vi "PID_Tuning.vi"() -> ()   [LabVIEW 2019]
uses:
  Shared VIs/ENPID/PID_Settings.ctl
  Shared VIs/ENPID/Gains.ctl
  Shared VIs/ENPID/NonLinearGainParams.ctl
  Shared VIs/ENPID/NonLinearGain.ctl
  Shared VIs/ENPID/DPartVariable.ctl
  Shared VIs/ENPID/VelocityEstimate.ctl
  Shared VIs/ENPID/OutputRange.ctl
  Shared VIs/ClusterType/RobotStateType.ctl
  Shared VIs/ModelSpecific/ETHMikeModel.ctl
  TrajectoryType.ctl
  Shared VIs/TypeDef_TDMS_States.ctl
  Shared VIs/ModelSpecific/TypeDefTachometerParam.ctl
  <vilib>/myRIO/Common/Instrument Driver Framework/myRIO v1.0/Encoder/typedefs/Encoder Signal Mode.ctl
  Shared VIs/ModelSpecific/ReadOnlyGlobalActions.ctl
  <vilib>/myRIO/Instrument Drivers/Onboard IO/AI/typedefs/AI Reference.ctl
  <vilib>/myRIO/Common/Instrument Driver Framework/Utilities/typedefs/myRIO Generic Hardware Reference.ctl
  <vilib>/myRIO/Common/Instrument Driver Framework/Utilities/typedefs/Hardware Version Enum.ctl
  <vilib>/myRIO/Common/Instrument Driver Framework/Utilities/typedefs/myRIO v1.0 Reference.ctl
  <vilib>/myRIO/Common/Instrument Driver Framework/Utilities/typedefs/Generic FPGA Reference.ctl
  <vilib>/myRIO/Common/Instrument Driver Framework/myRIO v1.0/AI/typedefs/AI Channels List.ctl
  <vilib>/myRIO/Common/Instrument Driver Framework/myRIO v1.0/AI/typedefs/AI Channels Enum.ctl
  <vilib>/myRIO/Common/Instrument Driver Framework/Utilities/typedefs/Analog Scaling Constants List.ctl
  <vilib>/myRIO/Common/Instrument Driver Framework/Utilities/typedefs/Analog Scaling Constants.ctl
  <vilib>/userDefined/High Color/nirio_resource_hc.ctl
  <vilib>/myRIO/Instrument Drivers/Onboard IO/AO/typedefs/AO Reference.ctl
  <vilib>/myRIO/Common/Instrument Driver Framework/myRIO v1.0/AO/typedefs/AO Channels List.ctl
  <vilib>/myRIO/Common/Instrument Driver Framework/myRIO v1.0/AO/typedefs/AO Channels Enum.ctl
  <vilib>/Platform/TimedLoop/XDataNode/timing_clust.ctl
  <vilib>/Platform/TimedLoop/XDataNode/nitl_modes.ctl
  <vilib>/Platform/TimedLoop/XDataNode/wakeup.ctl
  <vilib>/myRIO/Common/Instrument Driver Framework/myRIO v1.0/AI/vis/myRIO v1.1 Open AI.vi
  <vilib>/myRIO/Common/Instrument Driver Framework/myRIO v1.0/AO/vis/myRIO v1.1 Open AO.vi
  <vilib>/myRIO/Common/Instrument Driver Framework/Utilities/vis/Validate Channels.vi
  <vilib>/myRIO/Common/Instrument Driver Framework/myRIO v1.0/AI/vis/myRIO v1.0 Reserve AI.vi
  <vilib>/myRIO/Common/Instrument Driver Framework/myRIO v1.0/AO/vis/myRIO v1.0 Reserve AO.vi
  <vilib>/myRIO/Common/Instrument Driver Framework/myRIO v1.0/AO/vis/myRIO v1.0 Close AO.vi
  <vilib>/myRIO/Common/Instrument Driver Framework/myRIO v1.0/AI/vis/myRIO v1.0 Close AI.vi
  <vilib>/myRIO/Common/Instrument Driver Framework/myRIO v1.0/Encoder/vis/myRIO v1.0 Close Encoder.vi
  <vilib>/myRIO/Common/Instrument Driver Framework/myRIO v1.0/AI/vis/myRIO v1.0 Build MUX Configuration AI.vi
  <vilib>/myRIO/Common/Instrument Driver Framework/myRIO v1.0/Resource Manager/vis/myRIO v1.0 Reserve Channel List.vi
  <vilib>/myRIO/Common/Instrument Driver Framework/myRIO v1.0/AO/vis/myRIO v1.0 Build MUX Configuration AO.vi
  <vilib>/myRIO/Common/Instrument Driver Framework/myRIO v1.0/AO/vis/myRIO v1.0 Unreserve AO.vi
  <vilib>/myRIO/Common/Instrument Driver Framework/myRIO v1.0/AI/vis/myRIO v1.0 Unreserve AI.vi
  <vilib>/myRIO/Common/Instrument Driver Framework/myRIO v1.0/Encoder/vis/myRIO v1.0 Unreserve Encoder.vi
  <vilib>/myRIO/Common/Instrument Driver Framework/myRIO v1.0/Resource Manager/vis/myRIO v1.0 Reserve Channel.vi
  <vilib>/myRIO/Common/Instrument Driver Framework/myRIO v1.0/Resource Manager/vis/myRIO v1.0 Unreserve Channel.vi
  <vilib>/myRIO/Common/Instrument Driver Framework/myRIO v1.0/Resource Manager/vis/myRIO v1.0 Unreserve Channel List.vi
  <vilib>/myRIO/Common/Instrument Driver Framework/myRIO v1.0/Encoder/vis/myRIO v1.0 Build MUX Configuration Encoder.vi
  <vilib>/myRIO/Common/Instrument Driver Framework/myRIO v1.0/Resource Manager/vis/myRIO v1.0 Build Mutex Name.vi
  <vilib>/myRIO/Common/Instrument Driver Framework/myRIO v1.0/Resource Manager/vis/myRIO v1.0 Create Configuration List.vi
  <vilib>/Utility/VariantDataType/GetNumericInfo.vi
  <vilib>/Utility/error.llb/Error Cluster From Error Code.vi
  <vilib>/myRIO/Common/Instrument Driver Framework/myRIO v1.0/myRIO v1.1 Open.vi
  <vilib>/myRIO/Common/Instrument Driver Framework/myRIO v1.0/AO/vis/myRIO v1.0 Get Scaling Constants AO.vi
  <vilib>/myRIO/Common/Instrument Driver Framework/Utilities/vis/IO Manager.vi
  <vilib>/myRIO/Common/Instrument Driver Framework/Utilities/vis/Configuration Manager.vi
  <vilib>/myRIO/Common/Instrument Driver Framework/myRIO v1.0/myRIO v1.0 Close.vi
  <vilib>/myRIO/Common/Instrument Driver Framework/myRIO v1.0/AO/vis/myRIO v1.0 Write AO.vi
  <vilib>/myRIO/Common/Instrument Driver Framework/myRIO v1.0/AI/vis/myRIO v1.0 Get Scaling Constants AI.vi
  <vilib>/myRIO/Common/Instrument Driver Framework/myRIO v1.0/Encoder/vis/myRIO v1.0 Enable Encoder.vi
  <vilib>/myRIO/Common/Instrument Driver Framework/myRIO v1.0/Encoder/vis/myRIO v1.0 Shutdown Encoder.vi
  <vilib>/myRIO/Common/Instrument Driver Framework/myRIO v1.0/Resource Manager/vis/myRIO v1.0 Configure IO.vi
  <vilib>/myRIO/Instrument Drivers/Onboard IO/AO/vis/myRIO AO Open.xnode
  <vilib>/myRIO/Instrument Drivers/Onboard IO/AI/vis/myRIO AI Open.xnode
  <vilib>/platform/TimedLoop/XDataNode/XDataNode.xnode
  <vilib>/Platform/TimedLoop/XDataNode/XDNodeRunTimeDep.lvlib
  <vilib>/myRIO/Instrument Drivers/Onboard IO/AO/AO.lvlib
  <vilib>/myRIO/Instrument Drivers/Onboard IO/Encoder/Encoder.lvlib
  <vilib>/myRIO/Instrument Drivers/Onboard IO/AI/AI.lvlib
  <vilib>/addons/control/pid/NI_PID_pid.lvlib
  <vilib>/ptbypt/NI_PtbyPt.lvlib
panel:
  in  "Tachometer param":T1={"Offset [V]"=0.0, "Gain [deg/sV]"=130.0}
  out "Current Setpoint":dbl(graph)
  out "Control Output":dbl[][](graph)
  out "Control Output":cluster{"up":dbl, "ui":dbl, "ud":dbl, "u":dbl}(graph)
  out "Position Setpoint":dbl[][](graph)
  out "Velocity":cluster{"Velocity [deg/s]":dbl, dbl}(graph)
  out "Position":dbl(graph)
  out "u":cluster{"up":dbl, "ui":dbl, "ud":dbl, "u":dbl}
  out "TDMS States":T2
  in  "Trajectory Type":T3=enum."Sinus"
  in  "parameter source":T4=enum."ETH Mike #3" caption="From"
  in  "Load tuning parameter":bool caption="Boolean"
  in  "stop":bool
  out "RobotState":T5
  out "finished late":i16(graph)
  in  "PID Settings":T6={"Gains"={"K(e)"=0.0, "Kp"=0.800000011920929, "Ki"=0.0, "Kd"=0.003000000026077032}, "Non-linear gain"={"Non-linear gain P"=enum."off", "Non-linear gain I"=enum."off", "Non-linear gain D"=enum."off"}, "D-Part variable"=enum."process variable", "Velocity estimate dy/dt"=enum."external", "Anti reset windup"=TRUE, "I-Part error band"=inf, "Output range"={"output high"=0.0, "output low"=0.0}}
  in  "Target / HalfAmplitude  (deg)":dbl
  out "Current Setpoint [A]":dbl
  out "Position Setpoint [deg]":dbl
  in  "TDMS Storage File Input":string
  in  "Save data?":bool
  in  "Run":bool
  in  "Trajectory Duration (s)":dbl
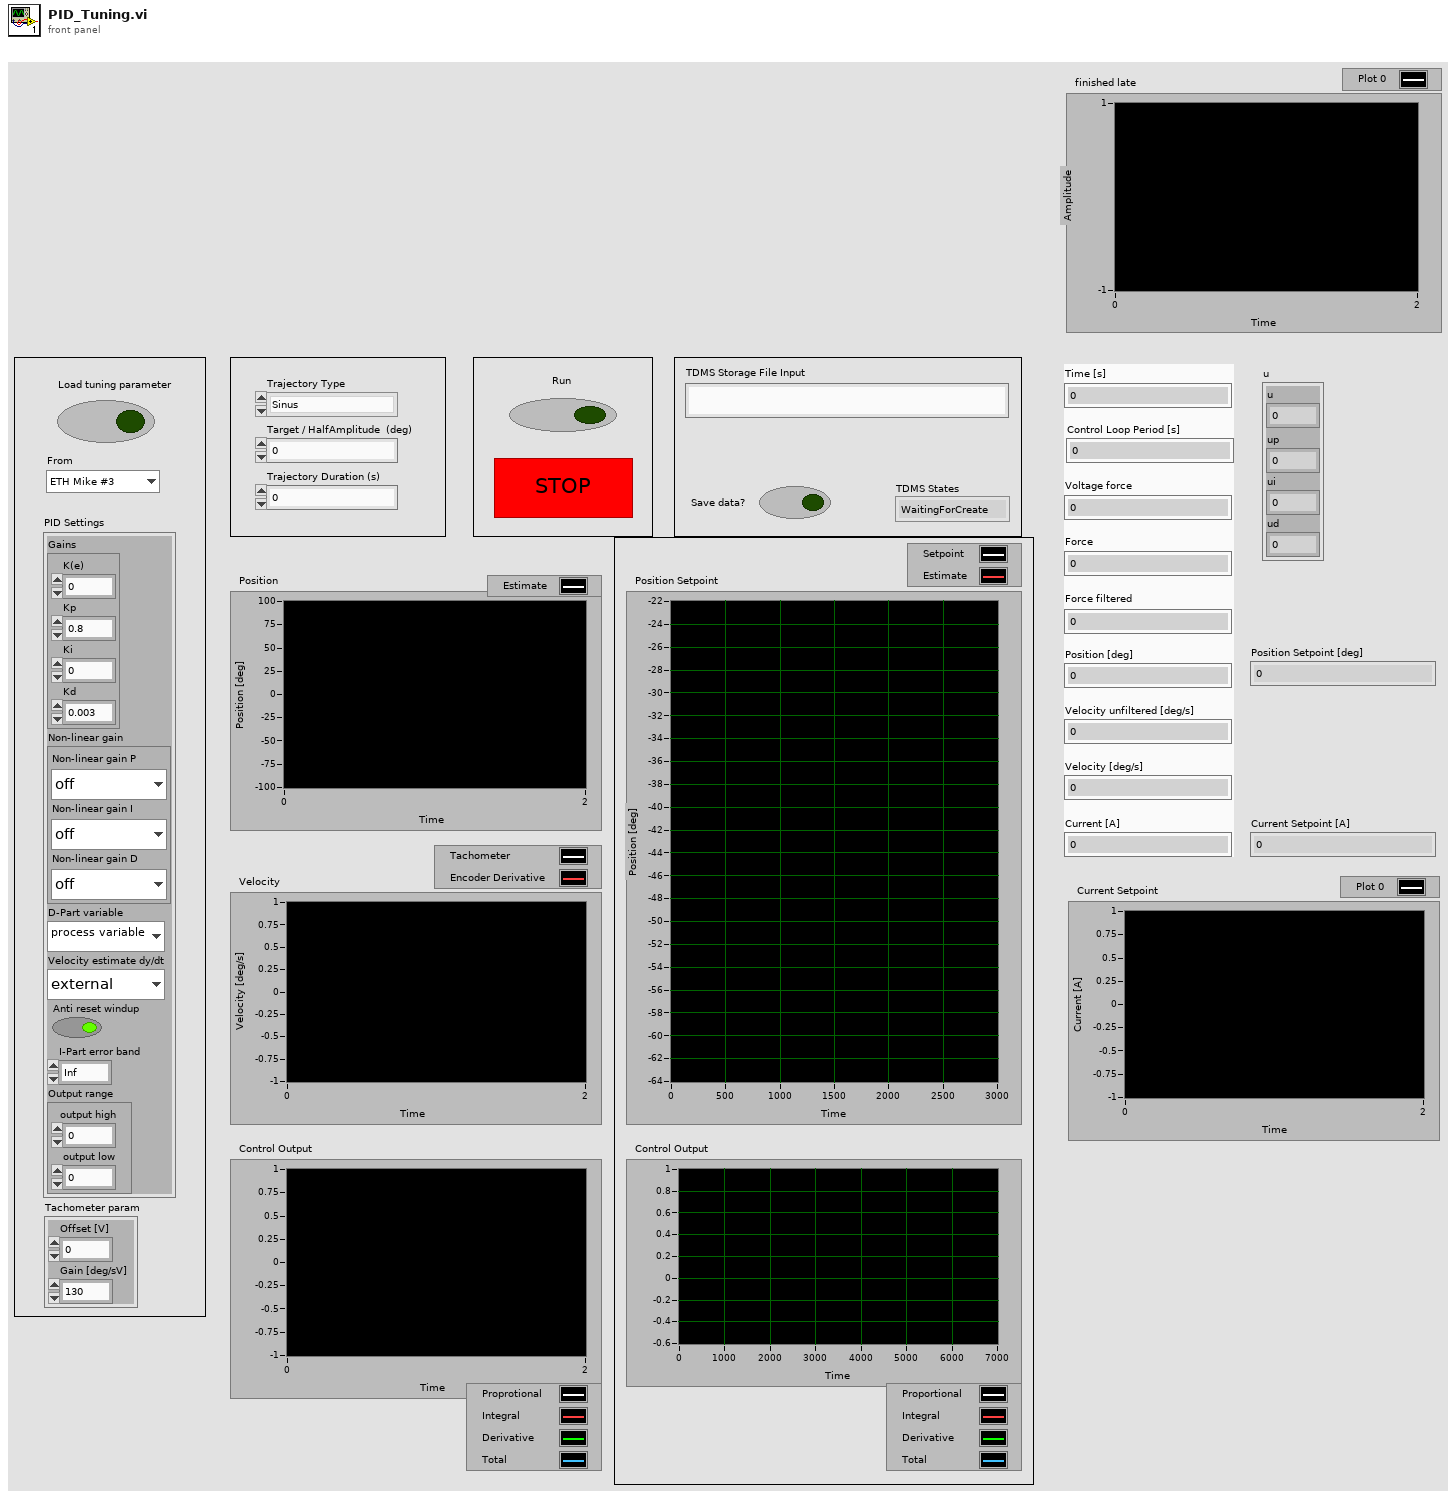
[diagram p1: front panel]
types:
  T1 = typedef "TypeDefTachometerParam.ctl" = cluster{"Offset [V]":dbl, "Gain [deg/sV]":dbl}
  T2 = typedef "TypeDef_TDMS_States.ctl" = enum16{"WaitingForCreate", "Create", "Buffering", "Flushing", "Write", "Close"}
  T3 = typedef "TrajectoryType.ctl" = enum16{"MinJerk", "Sinus", "Ramp"}
  T4 = typedef "ETHMikeModel.ctl" = enum16{"ETH Mike #1", "ETH Mike #2", "ETH Mike #3", "ETH Mike #4", "ETH MIKE #5"}
  T5 = typedef "RobotStateType.ctl" = cluster{"Time [s]":dbl, "Voltage force":dbl, "Force":dbl, "Force filtered":dbl, "Position [deg]":dbl, "Velocity unfiltered [deg/s]":dbl, "Velocity [deg/s]":dbl, "Current [A]":dbl, "Control Loop Period [s]":dbl}
  T6 = typedef "PID_Settings.ctl" = cluster{"Gains":T7, "Non-linear gain":T8, "D-Part variable":T10, "Velocity estimate dy/dt":T11, "Anti reset windup":bool, "I-Part error band":dbl, "Output range":T12}
  T7 = typedef "Gains.ctl" = cluster{"K(e)":dbl, "Kp":dbl, "Ki":dbl, "Kd":dbl}
  T8 = typedef "NonLinearGainParams.ctl" = cluster{"Non-linear gain P":T9, "Non-linear gain I":T9, "Non-linear gain D":T9}
  T9 = typedef "NonLinearGain.ctl" = enum16{"exponential", "quadratic", "off"}
  T10 = typedef "DPartVariable.ctl" = enum16{"error", "process variable"}
  T11 = typedef "VelocityEstimate.ctl" = enum16{"derivative", "external"}
  T12 = typedef "OutputRange.ctl" = cluster{"output high":dbl, "output low":dbl}
  T13 = typedef "nirio_resource_hc.ctl" = tag
  T14 = typedef "Hardware Version Enum.ctl" = enum16{"Unknown", "myRIO-1900", "myRIO-1950", "roboRIO", "NI ELVIS RIO CM", "ELVIS III"}
  T15 = enum16{"open", "open or create", "create or replace", "create", "open (read-only)"}
  T16 = typedef "XDNodeRunTimeDep.lvlib/timing_clust.ctl" = cluster{"Expected End [f-1]":u64, "Actual End [f-1]":u64, "Finished Late? [f-1]":bool, "Expected End [i-1]":u64, "Actual End [i-1]":u64, "Finished Late? [i-1]":bool, "Expected Start [i]":u64, "Actual Start [i]":u64, "Expected Start [f]":u64, "Actual Start [f]":u64, "Source Name":string, "Structure Name":string, "Period":i64, "Deadline":i64, "Offset":i64, "Start":i64, "Priority":i32, "Timeout":i32, "Mode":T17, "Wakeup Reason":T18, "Error":errorcluster, "Source Type":string, "Secondary Source Type":string, "Global End Time":u64, "Global Start Time":u64, "Frame Duration":u64, "Iteration Duration":u64, "Assigned CPU":i32, "I/O Scan Engine Mode":u32}
  T17 = typedef "XDNodeRunTimeDep.lvlib/nitl_modes.ctl" = enum32{"No Change", "Process missed periods, maintain original phase", "Discard missed periods, maintain original phase", "Process missed periods, ignore original phase", "Discard missed periods, ignore original phase"}
  T18 = typedef "XDNodeRunTimeDep.lvlib/wakeup.ctl" = enum32{"Normal", "Aborted", "Asynchronous wakeup", "Timing source error", "Timed loop error", "Timeout"}
  T19 = typedef "ReadOnlyGlobalActions.ctl" = enum16{"Initialize", "Read", "Write"}
  T20 = typedef "Encoder Signal Mode.ctl" = enum16{"Quadrature phase signal", "Step and direction signal"}
  T21 = typedef "AO.lvlib/AO Reference.ctl" = cluster{"myRIO Reference":T22, "AO Channel List":T25, "AO Scaling Constant List":T27}
  T22 = typedef "myRIO Generic Hardware Reference.ctl" = cluster{"myRIO Model":T14, "myRIO Hardware Reference":T23}
  T23 = typedef "myRIO v1.0 Reference.ctl" = cluster{"Generic FPGA Reference":T24, "Allow multiple opens":bool}
  T24 = typedef "Generic FPGA Reference.ctl" = refnum<k20>
  T25 = typedef "AO Channels List.ctl" = T26[]
  T26 = typedef "AO Channels Enum.ctl" = enum16{"Not Connected", "AudioOut/Left", "AudioOut/Right", "C/AO0", "C/AO1", "A/AO0", "A/AO1", "B/AO0", "B/AO1"}
  T27 = typedef "Analog Scaling Constants List.ctl" = T28[]
  T28 = typedef "Analog Scaling Constants.ctl" = cluster{"LSB Weight (Volts)":dbl, "Offset (Volts)":dbl, "Signed?":bool}
  T29 = typedef "Encoder.lvlib/Encoder Reference.ctl" = cluster{"myRIO Reference":T22, "Encoder Channels Enum":T30}
  T30 = typedef "Encoder Channels Enum.ctl" = enum16{"Not Connected", "C/ENC0", "C/ENC1", "A/ENC", "A/ENC0", "A/ENC1", "A/ENC2", "A/ENC3", "A/ENC4", "A/ENC5", "A/ENC6", "A/ENC7", "A/ENC8", "A/ENC9", "B/ENC", "B/ENC0", "B/ENC1", "B/ENC2", "B/ENC3", "B/ENC4", "B/ENC5", "B/ENC6", "B/ENC7", "B/ENC8", "B/ENC9", "DIO/ENC0", "DIO/ENC1", "DIO/ENC2", "DIO/ENC3", "DIO/ENC4"}
  T31 = typedef "AI.lvlib/AI Reference.ctl" = cluster{"myRIO Reference":T22, "AI Channels List":T32, "AI Scaling Constants List":T27}
  T32 = typedef "AI Channels List.ctl" = T33[]
  T33 = typedef "AI Channels Enum.ctl" = enum16{"Not Connected", "AudioIn/Left", "AudioIn/Right", "C/AI0", "C/AI1", "A/AI0", "A/AI1", "A/AI2", "A/AI3", "A/AI4", "A/AI5", "A/AI6", "A/AI7", "B/AI0", "B/AI1", "B/AI2", "B/AI3", "B/AI4", "B/AI5", "B/AI6", "B/AI7", "AI/AI0", "AI/AI1", "AI/AI2", "AI/AI3", "A/AI0 (DIFF)", "A/AI1 (DIFF)", "A/AI2 (DIFF)", "A/AI3 (DIFF)", "B/AI0 (DIFF)", "B/AI1 (DIFF)", "B/AI2 (DIFF)", "B/AI3 (DIFF)"}
  T34 = cluster{"Encoder":T29, "Tachometer":T31, "Motor Current Monitor":T31, "Force Sensor":T31}
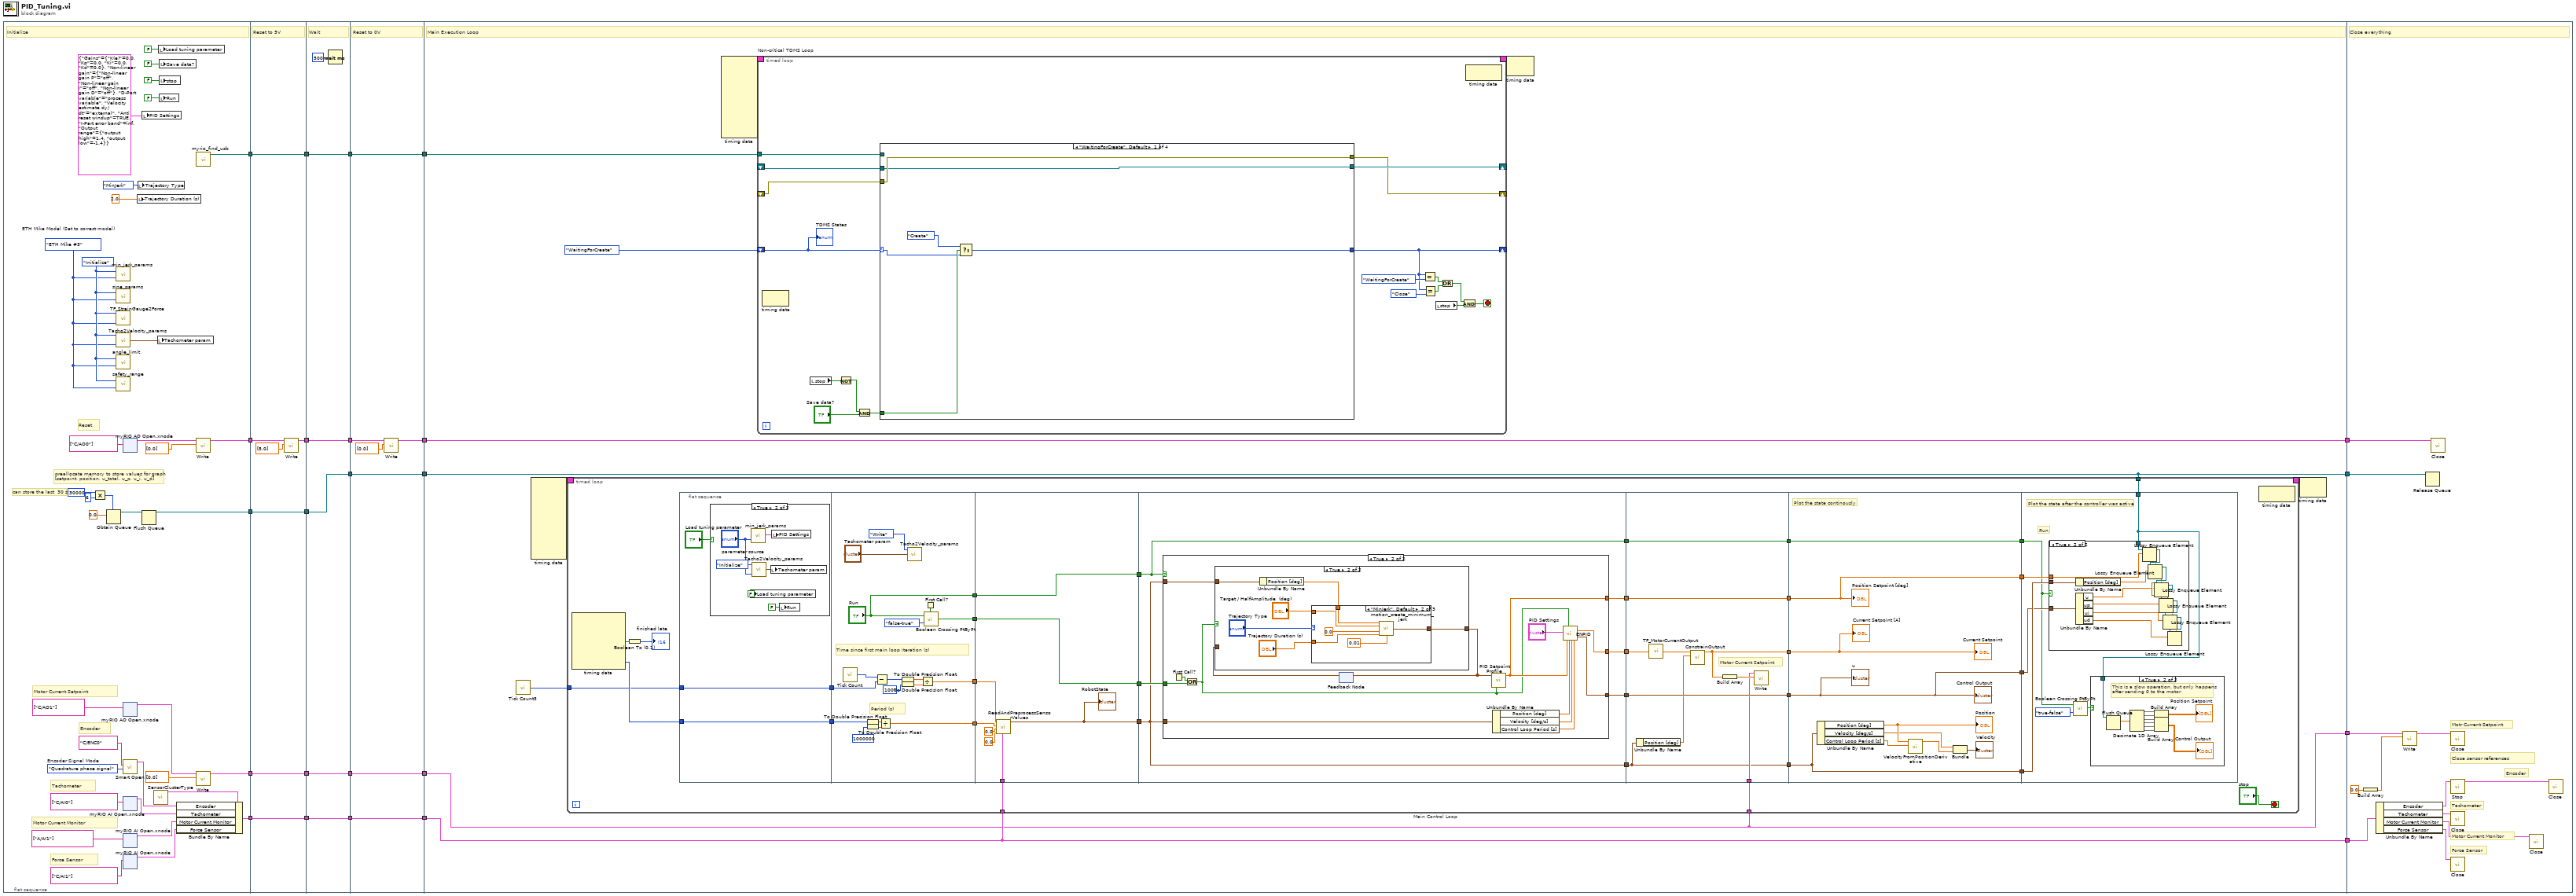
[diagram p0: block diagram]
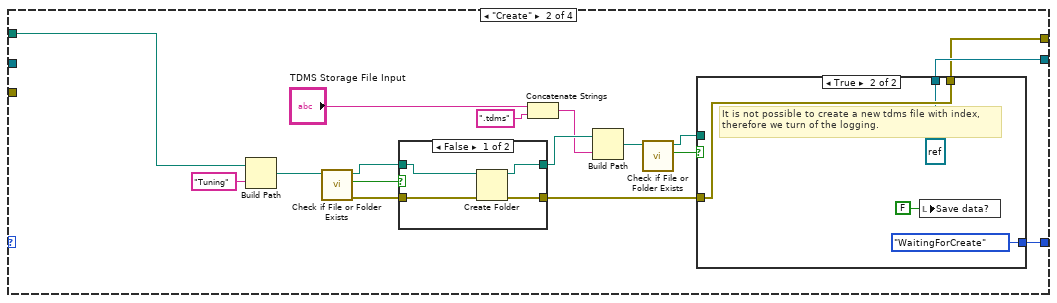
[diagram p2: hidden frame]
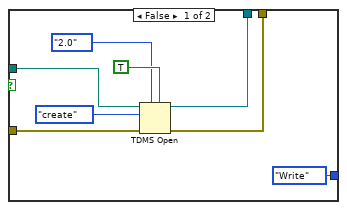
[diagram p3: hidden frame]
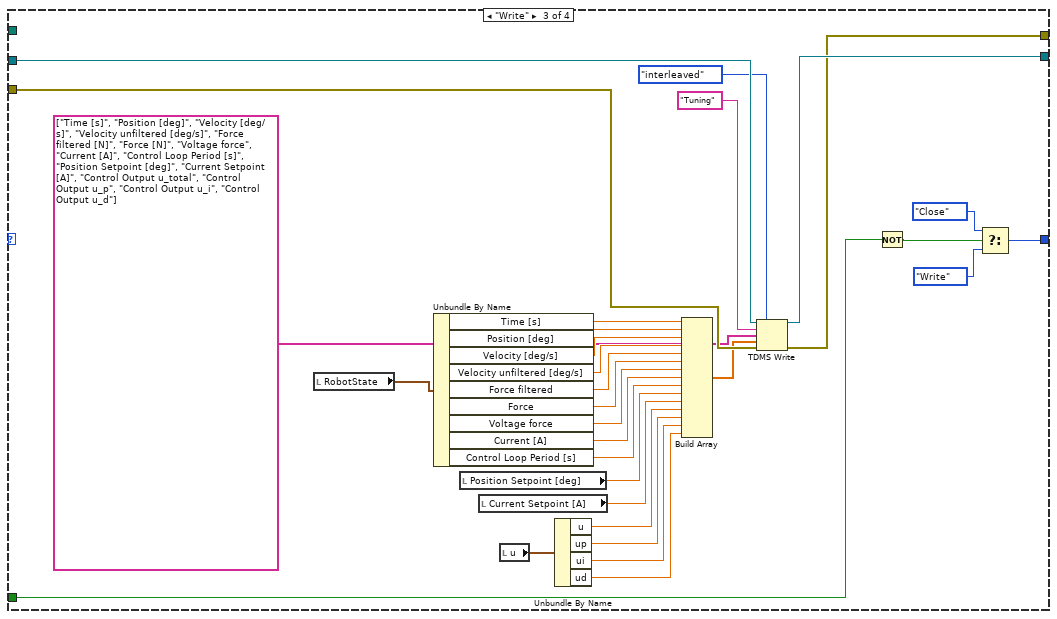
[diagram p5: hidden frame]
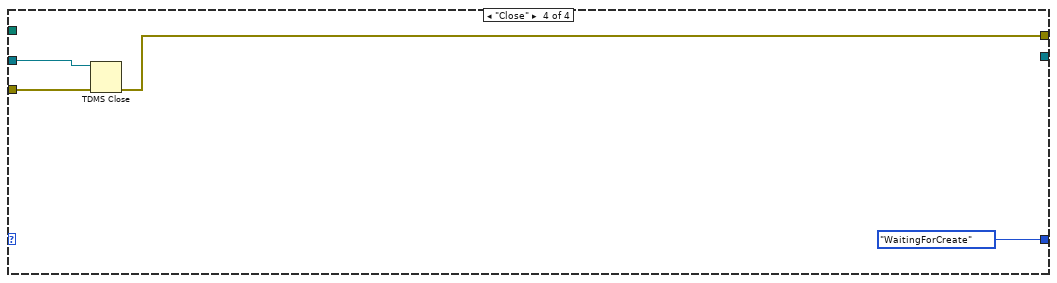
[diagram p6: hidden frame]
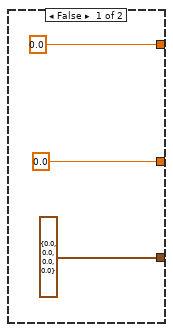
[diagram p8: hidden frame]
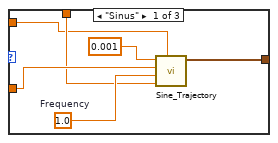
[diagram p10: hidden frame]
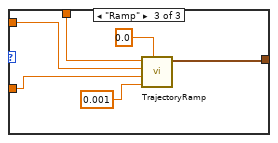
[diagram p11: hidden frame]
diagram:
  n1 = flat-sequence {
    tunnel: [w57] -> w24
    tunnel: [w53] -> w17
    tunnel: [w42] -> w13
    tunnel: [w41] -> w12
    tunnel: [w29] -> w2
    tunnel: w24 -> [w156]
    tunnel: [w155] -> w23
    tunnel: [w154] -> w18
    tunnel: w17 -> [w154]
    tunnel: [w153] -> w14
    tunnel: w13 -> [w153]
    tunnel: w12 -> [w152]
    tunnel: [w152] -> w11
    tunnel: [w151] -> w3
    tunnel: w2 -> [w151]
    tunnel: w23 -> [w163]
    tunnel: [w163] -> w22
    tunnel: [w161] -> w19
    tunnel: w18 -> [w161]
    tunnel: [w160] -> w15
    tunnel: w14 -> [w160]
    tunnel: w11 -> [w159]
    tunnel: [w159] -> w10
    tunnel: [w158] -> w4
    tunnel: w3 -> [w158]
    tunnel: w22 -> [w169]
    tunnel: [w168] -> w21
    tunnel: [w167] -> w20
    tunnel: w19 -> [w167]
    tunnel: [w166] -> w16
    tunnel: w15 -> [w166]
    tunnel: w10 -> [w165]
    tunnel: [w165] -> w9
    tunnel: [w164] -> w5
    tunnel: w4 -> [w164]
    tunnel: w21 -> [w178]
    tunnel: w20 -> [w179]
    tunnel: w16 -> [w176]
    tunnel: w9 -> [w175]
    tunnel: [w175] -> w8
    tunnel: [w176] -> w7
    tunnel: [w178] -> w6
    tunnel: w5 -> [w171]
    tunnel: [w171] -> w1
    tunnel: w8 -> [w463]
    tunnel: w7 -> [w457]
    tunnel: w6 -> [w456]
    tunnel: w1 -> [w455]
    frame #0 {
      w40 = ReadOnlyGlobalActions."Initialize" ("Action (Read)")
      w39 = ETHMikeModel."ETH Mike #3"  # ETH Mike Model (Set to correct model)
      w51 = Encoder_Signal_Mode."Quadrature phase signal"  # Encoder Signal Mode
      # "can store the last  30 s"
      # "preallocate memory to store values for graph\n[setpoint, position, u_total, u_p, u_i, u_d]"
      # "Force Sensor"
      # "Tachometer"
      # "Motor Current Monitor"
      # "Encoder"
      # "Motor Current Setpoint"
      # "Reset"
      # "Initialize"
      n2 = Multiply(x=30000 ("max queue size (-1, unlimited)"), y=6) -> (x*y=w26:i32)
      n3 = Obtain Queue(max queue size (-1, unlimited)=w26, element data type=0.0) -> (queue out=w30:refnum<queue>)  [unwired: 3 in, 2 out]
      n4 = call "min_jerk_params.vi"("Action (Read)"=w40, "ETH Mike Model"=w39) -> ()  [unwired: 17 in, 1 out]
      n5 = call "sine_params.vi"("Action (Read)"=w40, "ETH Mike Model"=w39) -> ()  [unwired: 17 in, 1 out]
      n6 = call "TF_StrainGauge2Force.vi"("Action (Read)"=w40, "ETH Mike Model"=w39) -> ()  [unwired: 3 in, 1 out]
      n7 = call "Tacho2Velocity_params.vi"("Action (Read)"=w40, "ETH Mike Model"=w39) -> ("Cluster"=w32:T1)  [unwired: 3 in]
      n8 = call "angle_limit.vi"("ETH Mike Model"=w39, "Action (Read)"=w40) -> ()  [unwired: 1 out]
      n9 = call "safety_range.vi"("ETH Mike Model"=w39, "Action (Read)"=w40) -> ()  [unwired: 1 out]
      n10 = xnode "myRIO AO Open.xnode"("Channel Names"=tag[] ["C/AO0"]) -> ("AO Ref Out"=w59:T21)  [unwired: 2 in, 1 out]
      n11 = xnode "myRIO AO Open.xnode"("Channel Names"=tag[] ["C/AO1"]) -> ("AO Ref Out"=w55:T21)  [unwired: 2 in, 1 out]
      n12 = call <vilib>:"Smart Open.vi"("Encoder Signal Mode"=w51, "Channel Name"=tag "C/ENC0") -> ("Encoder Ref Out"=w46:T29)  [unwired: 8 in, 1 out]
      n13 = xnode "myRIO AI Open.xnode"("Channel Names"=tag[] ["C/AI0"]) -> ("AI Ref Out"=w45:T31)  [unwired: 2 in, 1 out]
      n14 = xnode "myRIO AI Open.xnode"("Channel Names"=tag[] ["A/AI1"]) -> ("AI Ref Out"=w44:T31)  [unwired: 2 in, 1 out]
      n15 = xnode "myRIO AI Open.xnode"("Channel Names"=tag[] ["C/AI1"]) -> ("AI Ref Out"=w43:T31)  [unwired: 2 in, 1 out]
      n16 = local write "Trajectory Duration (s)"(2.0 ("Ramp Duration (s)")) -> ()
      n17 = local write "Trajectory Type"(TrajectoryType."MinJerk" ("Trajectory Type")) -> ()
      n18 = local write "PID Settings"(T6 {"Gains"={"K(e)"=0.0, "Kp"=0.0, "Ki"=0.0, "Kd"=0.0}, "Non-linear gain"={"Non-linear gain P"=enum."off", "Non-linear gain I"=enum."off", "Non-linear gain D"=enum."off"}, "D-Part variable"=enum."process variable", "Velocity estimate dy/dt"=enum."external", "Anti reset windup"=TRUE, "I-Part error band"=inf, "Output range"={"output high"=1.4, "output low"=-1.4}} ("PID Settings")) -> ()
      n19 = Flush Queue(queue=w30) -> (queue out=w29:refnum<queue>)  [unwired: 1 in, 2 out]
      n20 = call "SensorClusterType.vi"() -> ("Cluster"=w47:T34)  [unwired: 11 in]
      n21 = local write "Tachometer param"(w32) -> ()
      n22 = local write "Load tuning parameter"(FALSE ("Load tuning parameter")) -> ()
      n23 = local write "Save data?"(FALSE ("Save data?")) -> ()
      n24 = local write "stop"(FALSE ("stop")) -> ()
      n25 = local write "Run"(FALSE ("Run")) -> ()
      n26 = Bundle By Name(cluster=w47, "Encoder"=w46, "Tachometer"=w45, "Motor Current Monitor"=w44, "Force Sensor"=w43) -> (w42:T34)
      n27 = call <vilib>:"Write.vi"("Values"=dbl[] [0.0], "AO Ref In"=w59) -> ("AO Ref Out"=w57:T21)  [unwired: 7 in, 1 out]
      n28 = call <vilib>:"Write.vi"("Values"=dbl[] [0.0], "AO Ref In"=w55) -> ("AO Ref Out"=w41:T21)  [unwired: 7 in, 1 out]
      n29 = call "myrio_find_usb.vi"() -> ("Largest USB Partition Path"=w53:path)  [unwired: 9 in, 2 out]
    }
    frame #1 {
      # "Reset to 5V"
      n30 = call <vilib>:"Write.vi"("Values"=dbl[] [5.0], "AO Ref In"=w156) -> ("AO Ref Out"=w155:T21)  [unwired: 7 in, 1 out]
    }
    frame #2 {
      # "Wait"
      n31 = Wait (ms)(milliseconds to wait=500) -> ()  [unwired: 1 out]
    }
    frame #3 {
      # "Reset to 0V"
      n32 = call <vilib>:"Write.vi"("Values"=dbl[] [0.0], "AO Ref In"=w169) -> ("AO Ref Out"=w168:T21)  [unwired: 7 in, 1 out]
    }
    frame #4 {
      # "Main Execution Loop"
      n33 = call "Tick Count3"() -> ("Tick Count(mSec)"=w177:u32)
      n34 = node-c288() -> (w181:T16)  [unwired: 10 in]
      n35 = timed-loop "Main Control Loop" {
        timing: w181 -> [_]
        timing-out: [_] -> w180
        tunnel: w177 -> [w301]
        tunnel: w176 -> [w298]
        tunnel: w175 -> [w280]
        tunnel: w171 -> [w279]
        stop <- "stop" stop-if-true
        n36 = node-c288() -> (w308:bool, w302:i64)  [unwired: 1 in, 5 out]
        n37 = Boolean To (0,1)(Boolean=w308) -> (0, 1=→"finished late":i16)
        n38 = flat-sequence {
          tunnel: w301 -> [w311]
          tunnel: w302 -> [w312]
          tunnel: [w312] -> w296
          tunnel: [w311] -> w295
          tunnel: [w322] -> w307
          tunnel: ["Run"] -> w306
          tunnel: [w333] -> w303
          tunnel: [w325] -> w300
          tunnel: w296 -> [w327]
          tunnel: w295 -> [w326]
          tunnel: [w343] -> w305
          tunnel: [w344] -> w304
          tunnel: w307 -> [w343]
          tunnel: w306 -> [w344]
          tunnel: w298 -> [w342]
          tunnel: w303 -> [w339]
          tunnel: w300 -> [w338]
          tunnel: [w337] -> w299
          tunnel: [w349] -> w290
          tunnel: w305 -> [w350]
          tunnel: w304 -> [w345]
          tunnel: [w348] -> w289
          tunnel: w299 -> [w348]
          tunnel: [w347] -> w287
          tunnel: [w346] -> w285
          tunnel: [w345] -> w283
          tunnel: w290 -> [w399]
          tunnel: w289 -> [w395]
          tunnel: [w395] -> w288
          tunnel: w287 -> [w402]
          tunnel: [w402] -> w286
          tunnel: w285 -> [w401]
          tunnel: [w401] -> w284
          tunnel: w283 -> [w400]
          tunnel: [w400] -> w282
          tunnel: [w393] -> w281
          tunnel: w280 -> [w396]
          tunnel: w288 -> [w410]
          tunnel: w286 -> [w411]
          tunnel: w284 -> [w405]
          tunnel: w282 -> [w412]
          tunnel: [w412] -> w294
          tunnel: [w411] -> w293
          tunnel: [w410] -> w292
          tunnel: [w405] -> w291
          tunnel: w281 -> [w406]
          tunnel: w291 -> [w415]
          tunnel: w292 -> [w417]
          tunnel: w293 -> [w418]
          tunnel: w294 -> [w414]
          tunnel: w279 -> [w413]
          frame #0 {
            n39 = case shown="True" "Load tuning parameter" {
              frame False {
              }
              frame True {
                n40 = local write "Load tuning parameter"(FALSE ("Load parameter")) -> ()
                n41 = call "min_jerk_params.vi"("ETH Mike Model"="parameter source") -> ("PID Settings"=w316:T6)  [unwired: 18 in]
                n42 = call "Tacho2Velocity_params.vi"("Action (Read)"=ReadOnlyGlobalActions."Initialize", "ETH Mike Model"="parameter source") -> ("Cluster"=w314:T1)  [unwired: 3 in]
                n43 = local write "Tachometer param"(w314) -> ()
                n44 = local write "PID Settings"(w316) -> ()
                n45 = local write "Run"(FALSE ("Run")) -> ()
              }
            }
          }
          frame #1 {
            # "Time since first main loop iteration (s)"
            # "Period (s)"
            n46 = call "Tick Count"() -> ("Tick Count(mSec)"=w328:u32)
            n47 = To Double Precision Float(number=w327) -> (double precision float=w334:dbl)
            n48 = To Double Precision Float(number=1000000) -> (double precision float=w335:dbl)
            n49 = Subtract(x=w328, y=w326) -> (x-y=w331:u32)
            n50 = Divide(x=w334, y=w335) -> (x/y=w333:dbl)
            n51 = To Double Precision Float(number=w331) -> (double precision float=w329:dbl)
            n52 = To Double Precision Float(number=u32 1000 ("y")) -> (double precision float=w330:dbl)
            n53 = call "Tacho2Velocity_params.vi"("Action (Read)"=ReadOnlyGlobalActions."Write", "Tachometer param input"="Tachometer param") -> ()  [unwired: 3 in, 1 out]
            n54 = Divide(x=w329, y=w330) -> (x/y=w325:dbl)
            n55 = First Call?() -> (First Call?: T/F=w320:bool)
            n56 = call <vilib>:"Boolean Crossing PtByPt.vi"("initialize"=w320, "direction"=enum16{"either", "false-true", "true-false"}."false-true", "input"="Run") -> ("crossing"=w322:bool)
          }
          frame #2 {
            n57 = call "ReadAndPreprocessSensorValues.vi"("Sensor References"=w342, "Force_calib_value"=0.0, "Velocity_calib_value"=0.0, "Control Loop Period [s]"=w339, "Time [s]"=w338) -> ("RobotStateType"=w337:T5)  [unwired: 6 in]
            "RobotState" <- w337
          }
          frame #3 {
            n58 = case shown="True" w345 {
              tunnel: w350 -> [_ w364]
              tunnel: [0.0 ("u") w355] -> w349
              tunnel: w348 -> [_ w363]
              tunnel: w348 -> [_ w359]
              tunnel: [0.0 ("setpoint") w357] -> w347
              tunnel: [cluster{"up":dbl, "ui":dbl, "ud":dbl, "u":dbl} {"up"=0.0, "ui"=0.0, "ud"=0.0, "u"=0.0} ("u") w354] -> w346
              frame False {
              }
              frame True {
                n59 = First Call?() -> (First Call?: T/F=w365:bool)
                n60 = Or(x=w365, y=w364) -> (x .or. y?=w356:bool)
                n61 = feedback #1() -> (w366:cluster{"time (s)":dbl, "setpoint":dbl}[])  [unwired: 1 in]
                n62 = case shown="True" w356 {
                  tunnel: [w368 w374] -> w367
                  tunnel: w366 -> [w368 _]
                  tunnel: w359 -> [_ w371]
                  frame False {
                  }
                  frame True {
                    n63 = Unbundle By Name(w371) -> ("Position [deg]"=w370:dbl)
                    n64 = case shown="\"MinJerk\", Default" "Trajectory Type" {
                      tunnel: [w377 w386 w392] -> w374
                      tunnel: "Trajectory Duration (s)" -> [w378 w383 w391]
                      tunnel: "Target / HalfAmplitude  (deg)" -> [w375 w382 w390]
                      tunnel: w370 -> [w376 w381 w389]
                      frame "Sinus" {
                        w379 = 1.0  # Frequency
                        n65 = call "Sine_Trajectory.vi"("Amplitude"=w375, "Middle Position"=w376, "Cycles"=w379, "Duration (s)"=w378, "Sampling Period (s)"=0.001) -> ("Profile"=w377:cluster{"time (s)":dbl, "setpoint":dbl}[])  [unwired: 6 in]
                      }
                      frame "MinJerk", Default {
                        n66 = call "motion_create_minimum_jerk.vi"("Initial Position"=w381, "Final Position"=w382, "Initial Time [s]"=0.0, "Final Time [s]"=w383, "Delta Time [s]"=0.01) -> ("Profile"=w386:cluster{"time (s)":dbl, "setpoint":dbl}[])  [unwired: 10 in]
                      }
                      frame "Ramp" {
                        n67 = call "TrajectoryRamp.vi"("Initial Time (s)"=0.0, "Period (s)"=0.001, "Ramp Duration (s)"=w391, "Final Position (deg)"=w390, "Initial Position (deg)"=w389) -> ("Profile 2"=w392:cluster{"time (s)":dbl, "setpoint":dbl}[])  [unwired: 6 in]
                      }
                    }
                  }
                }
                n68 = feedback-in #1(w367) -> ()
                n69 = call <vilib>:"PID Setpoint Profile.vi"("reinitialize? (F)"=w356, "setpoint profile"=w367) -> ("setpoint"=w357:dbl)  [unwired: 4 in, 3 out]
                n70 = Unbundle By Name(w363) -> ("Position [deg]"=w362:dbl, "Velocity [deg/s]"=w361:dbl, "Control Loop Period [s]"=w360:dbl)
                n71 = call "ENPID.vi"("PID Settings"="PID Settings", "r"=w357, "Reset?"=w356, "y"=w362, "dy/dt"=w361, "dt (s)"=w360) -> (15:"u"=w355:dbl, 18:"u"=w354:cluster{"u":dbl, "up":dbl, "ui":dbl, "ud":dbl})  [unwired: 12 in]
              }
            }
          }
          frame #4 {
            # "Motor Current Setpoint"
            n72 = Unbundle By Name(w395) -> ("Position [deg]"=w394:dbl)
            n73 = call "TF_MotorCurrentOutput.vi"("Motor Current Setpoint [A]"=w399) -> ("Motor Current Setpoint [V]"=w398:dbl)
            n74 = call "ConstrainOutput.vi"("Position [deg]"=w394, "Motor Current Setpoint [V]"=w398) -> ("Motor Output"=w393:dbl)  [unwired: 9 in]
            n75 = Build Array(w393) -> (w397:dbl[])
            n76 = call <vilib>:"Write.vi"("Values"=w397, "AO Ref In"=w396) -> ()  [unwired: 7 in, 2 out]
          }
          frame #5 {
            # "Plot the state continously"
            n77 = Unbundle By Name(w410) -> ("Position [deg]"=w409:dbl, "Velocity [deg/s]"=w407:dbl, "Control Loop Period [s]"=w403:dbl)
            "Position" <- w409
            n78 = call "VelocityFromPositionDerivative.vi"("Control Loop Period [s]"=w403, "Position [deg]"=w409) -> ("Velocity"=w404:dbl)  [unwired: 9 in]
            n79 = Bundle("Velocity [deg/s]"=w407, "Velocity"=w404) -> (→"Velocity":cluster{"Velocity [deg/s]":dbl, "Velocity":dbl})  [unwired: 1 in]
            "Current Setpoint [A]" <- w406
            "Position Setpoint [deg]" <- w411
            "u" <- w405
            "Control Output" <- w405
            "Current Setpoint" <- w406
          }
          frame #6 {
            # "Plot the state after the controller was active"
            # "Run"
            n80 = case shown="True" w414 {
              tunnel: w418 -> [_ w435]
              tunnel: w417 -> [_ w438]
              tunnel: w415 -> [_ w437]
              tunnel: w413 -> [_ w436]
              frame False {
              }
              frame True {
                n81 = Unbundle By Name(w438) -> ("Position [deg]"=w429:dbl)
                n82 = Unbundle By Name(w437) -> ("u"=w423:dbl, "up"=w422:dbl, "ui"=w421:dbl, "ud"=w420:dbl)
                n83 = Lossy Enqueue Element(queue=w436, element=w435) -> (queue out=w434:refnum<queue>, error out=w428:errorcluster)  [unwired: 1 in, 2 out]
                n84 = Lossy Enqueue Element(queue=w434, element=w429, error in (no error)=w428) -> (queue out=w433:refnum<queue>, error out=w427:errorcluster)  [unwired: 2 out]
                n85 = Lossy Enqueue Element(queue=w433, element=w423, error in (no error)=w427) -> (queue out=w432:refnum<queue>, error out=w426:errorcluster)  [unwired: 2 out]
                n86 = Lossy Enqueue Element(queue=w432, element=w422, error in (no error)=w426) -> (queue out=w431:refnum<queue>, error out=w425:errorcluster)  [unwired: 2 out]
                n87 = Lossy Enqueue Element(queue=w431, element=w421, error in (no error)=w425) -> (queue out=w430:refnum<queue>, error out=w424:errorcluster)  [unwired: 2 out]
                n88 = Lossy Enqueue Element(queue=w430, element=w420, error in (no error)=w424) -> ()  [unwired: 4 out]
              }
            }
            n89 = call <vilib>:"Boolean Crossing PtByPt.vi"("direction"=enum16{"either", "false-true", "true-false"}."true-false", "input"=w414) -> ("crossing"=w419:bool)  [unwired: 1 in]
            n90 = case shown="True" w419 {
              tunnel: w413 -> [_ w448]
              frame False {
              }
              frame True {
                # "This is a slow operation, but only happens\nafter sending 0 to the motor"
                n91 = Flush Queue(queue=w448) -> (remaining elements=w445:dbl[])  [unwired: 1 in, 2 out]
                n92 = Decimate 1D Array(w445) -> (w447:dbl[], w446:dbl[], w443:dbl[], w442:dbl[], w441:dbl[], w440:dbl[])
                n93 = Build Array(w447, w446) -> (→"Position Setpoint":dbl[][])
                n94 = Build Array(w443, w442, w441, w440) -> (→"Control Output":dbl[][])
              }
            }
          }
        }
        n95 = node-c288() -> ()  [unwired: 1 in, 1 out]
      }
      n96 = node-c288() -> (w174:T16)  [unwired: 10 in]
      n97 = timed-loop "Non-critical TDMS Loop" {
        timing: w174 -> [_]
        timing-out: [_] -> w173
        shift-right: [w191] -> _
        shift-left: TypeDef_TDMS_States."WaitingForCreate" ("TDMS States") -> [w194]
        tunnel: w179 -> [w199]
        shift-right: [w198] -> _
        shift-left: _ -> [w195]
        shift-right: [w197] -> _
        shift-left: _ -> [w196]
        stop <- w188 stop-if-true
        n98 = node-c288() -> ()  [unwired: 1 in, 1 out]
        n99 = local read "stop"() -> (w183:bool)
        n100 = Not(x=w183) -> (.not. x?=w182:bool)
        n101 = And(x=w182, y="Save data?") -> (x .and. y?=w185:bool)
        n102 = case shown="\"WaitingForCreate\", Default" w194 {
          selector: w194 -> [w203 _ _ _]
          tunnel: w185 -> [w205 _ w266 _]
          tunnel: [w202 w222 w267 TypeDef_TDMS_States."WaitingForCreate" ("TDMS States")] -> w191
          tunnel: w199 -> [_ w208 _ _]
          tunnel: [w200 w221 w268 _] -> w198
          tunnel: [w201 w220 w247 w272] -> w197
          tunnel: w196 -> [w201 _ w270 w273]
          tunnel: w195 -> [w200 _ w269 w274]
          frame "WaitingForCreate", Default {
            n103 = Select(t=TypeDef_TDMS_States."Create" ("TDMS States"), s=w205, f=w203) -> (s? t:f=w202:T2)
          }
          frame "Create" {
            n104 = Build Path(base path=w208, name or relative path="Tuning") -> (appended path=w207:path)
            n105 = call <vilib>:"Check if File or Folder Exists.vi"("path"=w207) -> ("error out"=w217:errorcluster, "file or folder exists?"=w219:bool, "dup path"=w218:path)  [unwired: 8 in]
            n106 = case shown="False" w219 {
              tunnel: w218 -> [w238 w239]
              tunnel: [w237 w240] -> w212
              tunnel: w217 -> [w236 w240]
              tunnel: [w235 w239] -> w216
              frame False {
                n107 = Create Folder(path (use dialog)=w238, error in=w236) -> (created path=w235:path, error out=w237:errorcluster)  [unwired: 1 in, 1 out]
              }
              frame True {
              }
            }
            n108 = Concatenate Strings("TDMS Storage File Input", ".tdms") -> (w213:string)
            n109 = Build Path(base path=w216, name or relative path=w213) -> (appended path=w211:path)
            n110 = call <vilib>:"Check if File or Folder Exists.vi"("path"=w211) -> ("file or folder exists?"=w210:bool, "dup path"=w209:path)  [unwired: 8 in, 1 out]
            n111 = case shown="True" w210 {
              tunnel: [TypeDef_TDMS_States."Write" ("TDMS States") TypeDef_TDMS_States."WaitingForCreate" ("TDMS States")] -> w222
              tunnel: [w229 refnum<k34> refnum ("tdms file out")] -> w221
              tunnel: [w228 w232] -> w220
              tunnel: w212 -> [w224 w232]
              tunnel: w209 -> [w223 _]
              frame False {
                n112 = TDMS Open(5:TRUE, 7:enum16{"1.0", "2.0"}."2.0" ("file format version (2.0)"), 8:w224, 10:T15."create" ("operation (0:open)"), 11:w223) -> (0:w228:errorcluster, 3:w229:refnum<k34>)  [unwired: 2 in]
              }
              frame True {
                # "It is not possible to create a new tdms file with index,\ntherefore we turn of the logging."
                n113 = local write "Save data?"(FALSE ("Save data?")) -> ()
              }
            }
          }
          frame "Write" {
            n114 = local read "RobotState"() -> (w262:T5)
            n115 = Unbundle By Name(w262) -> ("Time [s]"=w261:dbl, "Position [deg]"=w260:dbl, "Velocity [deg/s]"=w259:dbl, "Velocity unfiltered [deg/s]"=w258:dbl, "Force filtered"=w254:dbl, "Force"=w253:dbl, "Voltage force"=w252:dbl, "Current [A]"=w251:dbl, "Control Loop Period [s]"=w250:dbl)
            n116 = local read "Position Setpoint [deg]"() -> (w249:dbl)
            n117 = local read "Current Setpoint [A]"() -> (w248:dbl)
            n118 = local read "u"() -> (w245:cluster{"up":dbl, "ui":dbl, "ud":dbl, "u":dbl})
            n119 = Unbundle By Name(w245) -> ("u"=w244:dbl, "up"=w243:dbl, "ui"=w242:dbl, "ud"=w241:dbl)
            n120 = Build Array(w261, w260, w259, w258, w254, w253, w252, w251, w250, w249, w248, w244, w243, w242, w241) -> (w264:dbl[])
            n121 = TDMS Write(0:w269, 1:enum16{"decimated", "interleaved"}."interleaved" ("data layout (0:decimated)"), 5:"Tuning" ("group name in (Untitled)"), 7:string[] ["Time [s]", "Position [deg]", "Velocity [deg/s]", "Velocity unfiltered [deg/s]", "Force filtered [N]", "Force [N]", "Voltage force", "Current [A]", "Control Loop Period [s]", "Position Setpoint [deg]", "Current Setpoint [A]", "Control Output u_total", "Control Output u_p", "Control Output u_i", "Control Output u_d"], 9:w264, 11:w270) -> (4:w268:refnum<k34>, 15:w247:errorcluster)  [unwired: 2 out]
            n122 = Not(x=w266) -> (.not. x?=w255:bool)
            n123 = Select(t=TypeDef_TDMS_States."Close" ("TDMS States"), s=w255, f=TypeDef_TDMS_States."Write" ("TDMS States")) -> (s? t:f=w267:T2)
          }
          frame "Close" {
            n124 = TDMS Close(8:w273, 11:w274) -> (0:w272:errorcluster)  [unwired: 1 out]
          }
        }
        n125 = Equal?(x=w191, y=TypeDef_TDMS_States."WaitingForCreate" ("TDMS States")) -> (x = y?=w190:bool)
        n126 = Equal?(x=w191, y=TypeDef_TDMS_States."Close" ("TDMS States")) -> (x = y?=w189:bool)
        n127 = local read "stop"() -> (w186:bool)
        n128 = Or(x=w190, y=w189) -> (x .or. y?=w187:bool)
        n129 = And(x=w187, y=w186) -> (x .and. y?=w188:bool)
        n130 = node-c288() -> ()  [unwired: 1 in, 1 out]
        "TDMS States" <- w194
      }
      n131 = node-c288(w173) -> ()  [unwired: 1 out]
      n132 = node-c288(w180) -> ()  [unwired: 1 out]
    }
    frame #5 {
      # "Close sensor references"
      # "Force Sensor"
      # "Tachometer"
      # "Motor Current Monitor"
      # "Encoder"
      # "Motr Current Setpoint"
      # "Close everything"
      n133 = Build Array(0.0) -> (w464:dbl[])
      n134 = Unbundle By Name(w457) -> ("Encoder"=w461:T29, "Tachometer"=w460:T31, "Motor Current Monitor"=w459:T31, "Force Sensor"=w458:T31)
      n135 = call <vilib>:"Write.vi"("Values"=w464, "AO Ref In"=w463) -> ("AO Ref Out"=w466:T21)  [unwired: 7 in, 1 out]
      n136 = Release Queue(queue=w455) -> ()  [unwired: 2 in, 3 out]
      n137 = call <vilib>:"Close.vi"("AO Ref In"=w456) -> ()  [unwired: 10 in, 1 out]
      n138 = call <vilib>:"Close.vi"("AO Ref In"=w466) -> ()  [unwired: 10 in, 1 out]
      n139 = call <vilib>:"Stop.vi"("Encoder Ref In"=w461) -> ("Encoder Ref Out"=w462:T29)  [unwired: 9 in, 1 out]
      n140 = call <vilib>:"Close.vi"("AI Ref In"=w460) -> ()  [unwired: 10 in, 1 out]
      n141 = call <vilib>:"Close.vi"("AI Ref In"=w458) -> ()  [unwired: 10 in, 1 out]
      n142 = call <vilib>:"Close.vi"("AI Ref In"=w459) -> ()  [unwired: 10 in, 1 out]
      n143 = call <vilib>:"Close.vi"("Encoder Ref In"=w462) -> ()  [unwired: 10 in, 1 out]
    }
  }
